vi "Ammeter Measure (Poly).vi"   [LabVIEW 2016, in "Hall Effect Library.lvlib"]
uses:
  Hall Effect Library.lvlib
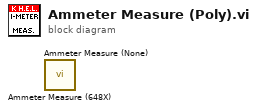
[diagram p0: block diagram]
diagram:
  n1 = call "Ammeter Measure (648X).vi"() -> ()  [unwired: 9 in, 3 out]
  n2 = call "Ammeter Measure (None).vi"() -> ()  [unwired: 9 in, 3 out]
